vi "App - analyze RUS V6.vi"() -> ()   [LabVIEW 2015] (continued)
"z(0)"=0.0+0.0i, "radius"=0.0}}, "timestamp(min)"=2140.5666666701436, "timestamp"=timestamp(3493856255 s since 1904-01-01), "Magn Field(T)"=0.0}, {"temperature"=14.643, "lorentzian"={"Amplitude"=0.0, "omega(0)"=0.0, "Gamma"=0.0, "phase"=0.0, "Q"=0.0, "Norm  Ampl"=0.0, "z (inf)"=0.0+0.0i, "4corners"={"z (-pi/2)"=0.0+0.0i, "z(inf)"=0.0+0.0i, "z (pi/2)"=0.0+0.0i, "z center"=0.0+0.0i, "z(0)"=0.0+0.0i, "radius"=0.0}}, "timestamp(min)"=2141.89999999851, "timestamp"=timestamp(3493856335 s since 1904-01-01), "Magn Field(T)"=0.0}, {"temperature"=14.643, "lorentzian"={"Amplitude"=0.0, "omega(0)"=0.0, "Gamma"=0.0, "phase"=0.0, "Q"=0.0, "Norm  Ampl"=0.0, "z (inf)"=0.0+0.0i, "4corners"={"z (-pi/2)"=0.0+0.0i, "z(inf)"=0.0+0.0i, "z (pi/2)"=0.0+0.0i, "z center"=0.0+0.0i, "z(0)"=0.0+0.0i, "radius"=0.0}}, "timestamp(min)"=2143.2166666686535, "timestamp"=timestamp(3493856414 s since 1904-01-01), "Magn Field(T)"=0.0}, {"temperature"=14.638, "lorentzian"={"Amplitude"=0.0, "omega(0)"=0.0, "Gamma"=0.0, "phase"=0.0, "Q"=0.0, "Norm  Ampl"=0.0, "z (inf)"=0.0+0.0i, "4corners"={"z (-pi/2)"=0.0+0.0i, "z(inf)"=0.0+0.0i, "z (pi/2)"=0.0+0.0i, "z center"=0.0+0.0i, "z(0)"=0.0+0.0i, "radius"=0.0}}, "timestamp(min)"=2144.5333333313465, "timestamp"=timestamp(3493856493 s since 1904-01-01), "Magn Field(T)"=0.0}, {"temperature"=14.634, "lorentzian"={"Amplitude"=0.0, "omega(0)"=0.0, "Gamma"=0.0, "phase"=0.0, "Q"=0.0, "Norm  Ampl"=0.0, "z (inf)"=0.0+0.0i, "4corners"={"z (-pi/2)"=0.0+0.0i, "z(inf)"=0.0+0.0i, "z (pi/2)"=0.0+0.0i, "z center"=0.0+0.0i, "z(0)"=0.0+0.0i, "radius"=0.0}}, "timestamp(min)"=2145.8666666671634, "timestamp"=timestamp(3493856573 s since 1904-01-01), "Magn Field(T)"=0.0}, {"temperature"=14.63, "lorentzian"={"Amplitude"=0.0, "omega(0)"=0.0, "Gamma"=0.0, "phase"=0.0, "Q"=0.0, "Norm  Ampl"=0.0, "z (inf)"=0.0+0.0i, "4corners"={"z (-pi/2)"=0.0+0.0i, "z(inf)"=0.0+0.0i, "z (pi/2)"=0.0+0.0i, "z center"=0.0+0.0i, "z(0)"=0.0+0.0i, "radius"=0.0}}, "timestamp(min)"=2147.183333337307, "timestamp"=timestamp(3493856652 s since 1904-01-01), "Magn Field(T)"=0.0}, {"temperature"=14.628, "lorentzian"={"Amplitude"=0.0, "omega(0)"=0.0, "Gamma"=0.0, "phase"=0.0, "Q"=0.0, "Norm  Ampl"=0.0, "z (inf)"=0.0+0.0i, "4corners"={"z (-pi/2)"=0.0+0.0i, "z(inf)"=0.0+0.0i, "z (pi/2)"=0.0+0.0i, "z center"=0.0+0.0i, "z(0)"=0.0+0.0i, "radius"=0.0}}, "timestamp(min)"=2148.5166666656733, "timestamp"=timestamp(3493856732 s since 1904-01-01), "Magn Field(T)"=0.0}, {"temperature"=14.626, "lorentzian"={"Amplitude"=0.0, "omega(0)"=0.0, "Gamma"=0.0, "phase"=0.0, "Q"=0.0, "Norm  Ampl"=0.0, "z (inf)"=0.0+0.0i, "4corners"={"z (-pi/2)"=0.0+0.0i, "z(inf)"=0.0+0.0i, "z (pi/2)"=0.0+0.0i, "z center"=0.0+0.0i, "z(0)"=0.0+0.0i, "radius"=0.0}}, "timestamp(min)"=2149.833333335817, "timestamp"=timestamp(3493856811 s since 1904-01-01), "Magn Field(T)"=0.0}, {"temperature"=14.618, "lorentzian"={"Amplitude"=0.0, "omega(0)"=0.0, "Gamma"=0.0, "phase"=0.0, "Q"=0.0, "Norm  Ampl"=0.0, "z (inf)"=0.0+0.0i, "4corners"={"z (-pi/2)"=0.0+0.0i, "z(inf)"=0.0+0.0i, "z (pi/2)"=0.0+0.0i, "z center"=0.0+0.0i, "z(0)"=0.0+0.0i, "radius"=0.0}}, "timestamp(min)"=2151.14999999851, "timestamp"=timestamp(3493856890 s since 1904-01-01), "Magn Field(T)"=0.0}, {"temperature"=14.618, "lorentzian"={"Amplitude"=0.0, "omega(0)"=0.0, "Gamma"=0.0, "phase"=0.0, "Q"=0.0, "Norm  Ampl"=0.0, "z (inf)"=0.0+0.0i, "4corners"={"z (-pi/2)"=0.0+0.0i, "z(inf)"=0.0+0.0i, "z (pi/2)"=0.0+0.0i, "z center"=0.0+0.0i, "z(0)"=0.0+0.0i, "radius"=0.0}}, "timestamp(min)"=2152.4666666686535, "timestamp"=timestamp(3493856969 s since 1904-01-01), "Magn Field(T)"=0.0}, {"temperature"=14.621, "lorentzian"={"Amplitude"=0.0, "omega(0)"=0.0, "Gamma"=0.0, "phase"=0.0, "Q"=0.0, "Norm  Ampl"=0.0, "z (inf)"=0.0+0.0i, "4corners"={"z (-pi/2)"=0.0+0.0i, "z(inf)"=0.0+0.0i, "z (pi/2)"=0.0+0.0i, "z center"=0.0+0.0i, "z(0)"=0.0+0.0i, "radius"=0.0}}, "timestamp(min)"=2153.8000000044703, "timestamp"=timestamp(3493857049 s since 1904-01-01), "Magn Field(T)"=0.0}, {"temperature"=14.616, "lorentzian"={"Amplitude"=0.0, "omega(0)"=0.0, "Gamma"=0.0, "phase"=0.0, "Q"=0.0, "Norm  Ampl"=0.0, "z (inf)"=0.0+0.0i, "4corners"={"z (-pi/2)"=0.0+0.0i, "z(inf)"=0.0+0.0i, "z (pi/2)"=0.0+0.0i, "z center"=0.0+0.0i, "z(0)"=0.0+0.0i, "radius"=0.0}}, "timestamp(min)"=2155.1166666671634, "timestamp"=timestamp(3493857128 s since 1904-01-01), "Magn Field(T)"=0.0}, {"temperature"=14.612, "lorentzian"={"Amplitude"=0.0, "omega(0)"=0.0, "Gamma"=0.0, "phase"=0.0, "Q"=0.0, "Norm  Ampl"=0.0, "z (inf)"=0.0+0.0i, "4corners"={"z (-pi/2)"=0.0+0.0i, "z(inf)"=0.0+0.0i, "z (pi/2)"=0.0+0.0i, "z center"=0.0+0.0i, "z(0)"=0.0+0.0i, "radius"=0.0}}, "timestamp(min)"=2156.433333337307, "timestamp"=timestamp(3493857207 s since 1904-01-01), "Magn Field(T)"=0.0}, {"temperature"=14.606, "lorentzian"={"Amplitude"=0.0, "omega(0)"=0.0, "Gamma"=0.0, "phase"=0.0, "Q"=0.0, "Norm  Ampl"=0.0, "z (inf)"=0.0+0.0i, "4corners"={"z (-pi/2)"=0.0+0.0i, "z(inf)"=0.0+0.0i, "z (pi/2)"=0.0+0.0i, "z center"=0.0+0.0i, "z(0)"=0.0+0.0i, "radius"=0.0}}, "timestamp(min)"=2157.75, "timestamp"=timestamp(3493857286 s since 1904-01-01), "Magn Field(T)"=0.0}, {"temperature"=14.604, "lorentzian"={"Amplitude"=0.0, "omega(0)"=0.0, "Gamma"=0.0, "phase"=0.0, "Q"=0.0, "Norm  Ampl"=0.0, "z (inf)"=0.0+0.0i, "4corners"={"z (-pi/2)"=0.0+0.0i, "z(inf)"=0.0+0.0i, "z (pi/2)"=0.0+0.0i, "z center"=0.0+0.0i, "z(0)"=0.0+0.0i, "radius"=0.0}}, "timestamp(min)"=2159.083333335817, "timestamp"=timestamp(3493857366 s since 1904-01-01), "Magn Field(T)"=0.0}, {"temperature"=14.604, "lorentzian"={"Amplitude"=0.0, "omega(0)"=0.0, "Gamma"=0.0, "phase"=0.0, "Q"=0.0, "Norm  Ampl"=0.0, "z (inf)"=0.0+0.0i, "4corners"={"z (-pi/2)"=0.0+0.0i, "z(inf)"=0.0+0.0i, "z (pi/2)"=0.0+0.0i, "z center"=0.0+0.0i, "z(0)"=0.0+0.0i, "radius"=0.0}}, "timestamp(min)"=2160.39999999851, "timestamp"=timestamp(3493857445 s since 1904-01-01), "Magn Field(T)"=0.0}, {"temperature"=14.606, "lorentzian"={"Amplitude"=0.0, "omega(0)"=0.0, "Gamma"=0.0, "phase"=0.0, "Q"=0.0, "Norm  Ampl"=0.0, "z (inf)"=0.0+0.0i, "4corners"={"z (-pi/2)"=0.0+0.0i, "z(inf)"=0.0+0.0i, "z (pi/2)"=0.0+0.0i, "z center"=0.0+0.0i, "z(0)"=0.0+0.0i, "radius"=0.0}}, "timestamp(min)"=2161.7166666686535, "timestamp"=timestamp(3493857524 s since 1904-01-01), "Magn Field(T)"=0.0}, {"temperature"=14.605, "lorentzian"={"Amplitude"=0.0, "omega(0)"=0.0, "Gamma"=0.0, "phase"=0.0, "Q"=0.0, "Norm  Ampl"=0.0, "z (inf)"=0.0+0.0i, "4corners"={"z (-pi/2)"=0.0+0.0i, "z(inf)"=0.0+0.0i, "z (pi/2)"=0.0+0.0i, "z center"=0.0+0.0i, "z(0)"=0.0+0.0i, "radius"=0.0}}, "timestamp(min)"=2163.0500000044703, "timestamp"=timestamp(3493857604 s since 1904-01-01), "Magn Field(T)"=0.0}, {"temperature"=14.606, "lorentzian"={"Amplitude"=0.0, "omega(0)"=0.0, "Gamma"=0.0, "phase"=0.0, "Q"=0.0, "Norm  Ampl"=0.0, "z (inf)"=0.0+0.0i, "4corners"={"z (-pi/2)"=0.0+0.0i, "z(inf)"=0.0+0.0i, "z (pi/2)"=0.0+0.0i, "z center"=0.0+0.0i, "z(0)"=0.0+0.0i, "radius"=0.0}}, "timestamp(min)"=2164.3666666671634, "timestamp"=timestamp(3493857683 s since 1904-01-01), "Magn Field(T)"=0.0}, {"temperature"=14.603, "lorentzian"={"Amplitude"=0.0, "omega(0)"=0.0, "Gamma"=0.0, "phase"=0.0, "Q"=0.0, "Norm  Ampl"=0.0, "z (inf)"=0.0+0.0i, "4corners"={"z (-pi/2)"=0.0+0.0i, "z(inf)"=0.0+0.0i, "z (pi/2)"=0.0+0.0i, "z center"=0.0+0.0i, "z(0)"=0.0+0.0i, "radius"=0.0}}, "timestamp(min)"=2165.683333337307, "timestamp"=timestamp(3493857762 s since 1904-01-01), "Magn Field(T)"=0.0}, {"temperature"=14.6, "lorentzian"={"Amplitude"=0.0, "omega(0)"=0.0, "Gamma"=0.0, "phase"=0.0, "Q"=0.0, "Norm  Ampl"=0.0, "z (inf)"=0.0+0.0i, "4corners"={"z (-pi/2)"=0.0+0.0i, "z(inf)"=0.0+0.0i, "z (pi/2)"=0.0+0.0i, "z center"=0.0+0.0i, "z(0)"=0.0+0.0i, "radius"=0.0}}, "timestamp(min)"=2167.0166666656733, "timestamp"=timestamp(3493857842 s since 1904-01-01), "Magn Field(T)"=0.0}, {"temperature"=14.601, "lorentzian"={"Amplitude"=0.0, "omega(0)"=0.0, "Gamma"=0.0, "phase"=0.0, "Q"=0.0, "Norm  Ampl"=0.0, "z (inf)"=0.0+0.0i, "4corners"={"z (-pi/2)"=0.0+0.0i, "z(inf)"=0.0+0.0i, "z (pi/2)"=0.0+0.0i, "z center"=0.0+0.0i, "z(0)"=0.0+0.0i, "radius"=0.0}}, "timestamp(min)"=2168.333333335817, "timestamp"=timestamp(3493857921 s since 1904-01-01), "Magn Field(T)"=0.0}, {"temperature"=14.595, "lorentzian"={"Amplitude"=0.0, "omega(0)"=0.0, "Gamma"=0.0, "phase"=0.0, "Q"=0.0, "Norm  Ampl"=0.0, "z (inf)"=0.0+0.0i, "4corners"={"z (-pi/2)"=0.0+0.0i, "z(inf)"=0.0+0.0i, "z (pi/2)"=0.0+0.0i, "z center"=0.0+0.0i, "z(0)"=0.0+0.0i, "radius"=0.0}}, "timestamp(min)"=2169.64999999851, "timestamp"=timestamp(3493858000 s since 1904-01-01), "Magn Field(T)"=0.0}, {"temperature"=14.592, "lorentzian"={"Amplitude"=0.0, "omega(0)"=0.0, "Gamma"=0.0, "phase"=0.0, "Q"=0.0, "Norm  Ampl"=0.0, "z (inf)"=0.0+0.0i, "4corners"={"z (-pi/2)"=0.0+0.0i, "z(inf)"=0.0+0.0i, "z (pi/2)"=0.0+0.0i, "z center"=0.0+0.0i, "z(0)"=0.0+0.0i, "radius"=0.0}}, "timestamp(min)"=2170.9833333343267, "timestamp"=timestamp(3493858080 s since 1904-01-01), "Magn Field(T)"=0.0}, {"temperature"=14.59, "lorentzian"={"Amplitude"=0.0, "omega(0)"=0.0, "Gamma"=0.0, "phase"=0.0, "Q"=0.0, "Norm  Ampl"=0.0, "z (inf)"=0.0+0.0i, "4corners"={"z (-pi/2)"=0.0+0.0i, "z(inf)"=0.0+0.0i, "z (pi/2)"=0.0+0.0i, "z center"=0.0+0.0i, "z(0)"=0.0+0.0i, "radius"=0.0}}, "timestamp(min)"=2172.3000000044703, "timestamp"=timestamp(3493858159 s since 1904-01-01), "Magn Field(T)"=0.0}, {"temperature"=14.588, "lorentzian"={"Amplitude"=0.0, "omega(0)"=0.0, "Gamma"=0.0, "phase"=0.0, "Q"=0.0, "Norm  Ampl"=0.0, "z (inf)"=0.0+0.0i, "4corners"={"z (-pi/2)"=0.0+0.0i, "z(inf)"=0.0+0.0i, "z (pi/2)"=0.0+0.0i, "z center"=0.0+0.0i, "z(0)"=0.0+0.0i, "radius"=0.0}}, "timestamp(min)"=2173.6166666671634, "timestamp"=timestamp(3493858238 s since 1904-01-01), "Magn Field(T)"=0.0}, {"temperature"=14.586, "lorentzian"={"Amplitude"=0.0, "omega(0)"=0.0, "Gamma"=0.0, "phase"=0.0, "Q"=0.0, "Norm  Ampl"=0.0, "z (inf)"=0.0+0.0i, "4corners"={"z (-pi/2)"=0.0+0.0i, "z(inf)"=0.0+0.0i, "z (pi/2)"=0.0+0.0i, "z center"=0.0+0.0i, "z(0)"=0.0+0.0i, "radius"=0.0}}, "timestamp(min)"=2174.9500000029802, "timestamp"=timestamp(3493858318 s since 1904-01-01), "Magn Field(T)"=0.0}, {"temperature"=14.583, "lorentzian"={"Amplitude"=0.0, "omega(0)"=0.0, "Gamma"=0.0, "phase"=0.0, "Q"=0.0, "Norm  Ampl"=0.0, "z (inf)"=0.0+0.0i, "4corners"={"z (-pi/2)"=0.0+0.0i, "z(inf)"=0.0+0.0i, "z (pi/2)"=0.0+0.0i, "z center"=0.0+0.0i, "z(0)"=0.0+0.0i, "radius"=0.0}}, "timestamp(min)"=2176.2666666656733, "timestamp"=timestamp(3493858397 s since 1904-01-01), "Magn Field(T)"=0.0}, {"temperature"=14.577, "lorentzian"={"Amplitude"=0.0, "omega(0)"=0.0, "Gamma"=0.0, "phase"=0.0, "Q"=0.0, "Norm  Ampl"=0.0, "z (inf)"=0.0+0.0i, "4corners"={"z (-pi/2)"=0.0+0.0i, "z(inf)"=0.0+0.0i, "z (pi/2)"=0.0+0.0i, "z center"=0.0+0.0i, "z(0)"=0.0+0.0i, "radius"=0.0}}, "timestamp(min)"=2177.60000000149, "timestamp"=timestamp(3493858477 s since 1904-01-01), "Magn Field(T)"=0.0}, {"temperature"=14.575, "lorentzian"={"Amplitude"=0.0, "omega(0)"=0.0, "Gamma"=0.0, "phase"=0.0, "Q"=0.0, "Norm  Ampl"=0.0, "z (inf)"=0.0+0.0i, "4corners"={"z (-pi/2)"=0.0+0.0i, "z(inf)"=0.0+0.0i, "z (pi/2)"=0.0+0.0i, "z center"=0.0+0.0i, "z(0)"=0.0+0.0i, "radius"=0.0}}, "timestamp(min)"=2178.916666664183, "timestamp"=timestamp(3493858556 s since 1904-01-01), "Magn Field(T)"=0.0}, {"temperature"=14.575, "lorentzian"={"Amplitude"=0.0, "omega(0)"=0.0, "Gamma"=0.0, "phase"=0.0, "Q"=0.0, "Norm  Ampl"=0.0, "z (inf)"=0.0+0.0i, "4corners"={"z (-pi/2)"=0.0+0.0i, "z(inf)"=0.0+0.0i, "z (pi/2)"=0.0+0.0i, "z center"=0.0+0.0i, "z(0)"=0.0+0.0i, "radius"=0.0}}, "timestamp(min)"=2180.2333333343267, "timestamp"=timestamp(3493858635 s since 1904-01-01), "Magn Field(T)"=0.0}, {"temperature"=14.572, "lorentzian"={"Amplitude"=0.0, "omega(0)"=0.0, "Gamma"=0.0, "phase"=0.0, "Q"=0.0, "Norm  Ampl"=0.0, "z (inf)"=0.0+0.0i, "4corners"={"z (-pi/2)"=0.0+0.0i, "z(inf)"=0.0+0.0i, "z (pi/2)"=0.0+0.0i, "z center"=0.0+0.0i, "z(0)"=0.0+0.0i, "radius"=0.0}}, "timestamp(min)"=2181.5666666701436, "timestamp"=timestamp(3493858715 s since 1904-01-01), "Magn Field(T)"=0.0}, {"temperature"=14.574, "lorentzian"={"Amplitude"=0.0, "omega(0)"=0.0, "Gamma"=0.0, "phase"=0.0, "Q"=0.0, "Norm  Ampl"=0.0, "z (inf)"=0.0+0.0i, "4corners"={"z (-pi/2)"=0.0+0.0i, "z(inf)"=0.0+0.0i, "z (pi/2)"=0.0+0.0i, "z center"=0.0+0.0i, "z(0)"=0.0+0.0i, "radius"=0.0}}, "timestamp(min)"=2182.8833333328366, "timestamp"=timestamp(3493858794 s since 1904-01-01), "Magn Field(T)"=0.0}, {"temperature"=14.57, "lorentzian"={"Amplitude"=0.0, "omega(0)"=0.0, "Gamma"=0.0, "phase"=0.0, "Q"=0.0, "Norm  Ampl"=0.0, "z (inf)"=0.0+0.0i, "4corners"={"z (-pi/2)"=0.0+0.0i, "z(inf)"=0.0+0.0i, "z (pi/2)"=0.0+0.0i, "z center"=0.0+0.0i, "z(0)"=0.0+0.0i, "radius"=0.0}}, "timestamp(min)"=2184.2000000029802, "timestamp"=timestamp(3493858873 s since 1904-01-01), "Magn Field(T)"=0.0}, {"temperature"=14.574, "lorentzian"={"Amplitude"=0.0, "omega(0)"=0.0, "Gamma"=0.0, "phase"=0.0, "Q"=0.0, "Norm  Ampl"=0.0, "z (inf)"=0.0+0.0i, "4corners"={"z (-pi/2)"=0.0+0.0i, "z(inf)"=0.0+0.0i, "z (pi/2)"=0.0+0.0i, "z center"=0.0+0.0i, "z(0)"=0.0+0.0i, "radius"=0.0}}, "timestamp(min)"=2185.5333333313465, "timestamp"=timestamp(3493858953 s since 1904-01-01), "Magn Field(T)"=0.0}, {"temperature"=14.576, "lorentzian"={"Amplitude"=0.0, "omega(0)"=0.0, "Gamma"=0.0, "phase"=0.0, "Q"=0.0, "Norm  Ampl"=0.0, "z (inf)"=0.0+0.0i, "4corners"={"z (-pi/2)"=0.0+0.0i, "z(inf)"=0.0+0.0i, "z (pi/2)"=0.0+0.0i, "z center"=0.0+0.0i, "z(0)"=0.0+0.0i, "radius"=0.0}}, "timestamp(min)"=2186.85000000149, "timestamp"=timestamp(3493859032 s since 1904-01-01), "Magn Field(T)"=0.0}, {"temperature"=14.575, "lorentzian"={"Amplitude"=0.0, "omega(0)"=0.0, "Gamma"=0.0, "phase"=0.0, "Q"=0.0, "Norm  Ampl"=0.0, "z (inf)"=0.0+0.0i, "4corners"={"z (-pi/2)"=0.0+0.0i, "z(inf)"=0.0+0.0i, "z (pi/2)"=0.0+0.0i, "z center"=0.0+0.0i, "z(0)"=0.0+0.0i, "radius"=0.0}}, "timestamp(min)"=2188.183333337307, "timestamp"=timestamp(3493859112 s since 1904-01-01), "Magn Field(T)"=0.0}, {"temperature"=14.567, "lorentzian"={"Amplitude"=0.0, "omega(0)"=0.0, "Gamma"=0.0, "phase"=0.0, "Q"=0.0, "Norm  Ampl"=0.0, "z (inf)"=0.0+0.0i, "4corners"={"z (-pi/2)"=0.0+0.0i, "z(inf)"=0.0+0.0i, "z (pi/2)"=0.0+0.0i, "z center"=0.0+0.0i, "z(0)"=0.0+0.0i, "radius"=0.0}}, "timestamp(min)"=2189.5, "timestamp"=timestamp(3493859191 s since 1904-01-01), "Magn Field(T)"=0.0}, {"temperature"=14.572, "lorentzian"={"Amplitude"=0.0, "omega(0)"=0.0, "Gamma"=0.0, "phase"=0.0, "Q"=0.0, "Norm  Ampl"=0.0, "z (inf)"=0.0+0.0i, "4corners"={"z (-pi/2)"=0.0+0.0i, "z(inf)"=0.0+0.0i, "z (pi/2)"=0.0+0.0i, "z center"=0.0+0.0i, "z(0)"=0.0+0.0i, "radius"=0.0}}, "timestamp(min)"=2190.8166666701436, "timestamp"=timestamp(3493859270 s since 1904-01-01), "Magn Field(T)"=0.0}, {"temperature"=14.571, "lorentzian"={"Amplitude"=0.0, "omega(0)"=0.0, "Gamma"=0.0, "phase"=0.0, "Q"=0.0, "Norm  Ampl"=0.0, "z (inf)"=0.0+0.0i, "4corners"={"z (-pi/2)"=0.0+0.0i, "z(inf)"=0.0+0.0i, "z (pi/2)"=0.0+0.0i, "z center"=0.0+0.0i, "z(0)"=0.0+0.0i, "radius"=0.0}}, "timestamp(min)"=2192.14999999851, "timestamp"=timestamp(3493859350 s since 1904-01-01), "Magn Field(T)"=0.0}, {"temperature"=14.568, "lorentzian"={"Amplitude"=0.0, "omega(0)"=0.0, "Gamma"=0.0, "phase"=0.0, "Q"=0.0, "Norm  Ampl"=0.0, "z (inf)"=0.0+0.0i, "4corners"={"z (-pi/2)"=0.0+0.0i, "z(inf)"=0.0+0.0i, "z (pi/2)"=0.0+0.0i, "z center"=0.0+0.0i, "z(0)"=0.0+0.0i, "radius"=0.0}}, "timestamp(min)"=2193.4666666686535, "timestamp"=timestamp(3493859429 s since 1904-01-01), "Magn Field(T)"=0.0}, {"temperature"=14.564, "lorentzian"={"Amplitude"=0.0, "omega(0)"=0.0, "Gamma"=0.0, "phase"=0.0, "Q"=0.0, "Norm  Ampl"=0.0, "z (inf)"=0.0+0.0i, "4corners"={"z (-pi/2)"=0.0+0.0i, "z(inf)"=0.0+0.0i, "z (pi/2)"=0.0+0.0i, "z center"=0.0+0.0i, "z(0)"=0.0+0.0i, "radius"=0.0}}, "timestamp(min)"=2194.7833333313465, "timestamp"=timestamp(3493859508 s since 1904-01-01), "Magn Field(T)"=0.0}, {"temperature"=14.565, "lorentzian"={"Amplitude"=0.0, "omega(0)"=0.0, "Gamma"=0.0, "phase"=0.0, "Q"=0.0, "Norm  Ampl"=0.0, "z (inf)"=0.0+0.0i, "4corners"={"z (-pi/2)"=0.0+0.0i, "z(inf)"=0.0+0.0i, "z (pi/2)"=0.0+0.0i, "z center"=0.0+0.0i, "z(0)"=0.0+0.0i, "radius"=0.0}}, "timestamp(min)"=2196.1166666671634, "timestamp"=timestamp(3493859588 s since 1904-01-01), "Magn Field(T)"=0.0}, {"temperature"=14.561, "lorentzian"={"Amplitude"=0.0, "omega(0)"=0.0, "Gamma"=0.0, "phase"=0.0, "Q"=0.0, "Norm  Ampl"=0.0, "z (inf)"=0.0+0.0i, "4corners"={"z (-pi/2)"=0.0+0.0i, "z(inf)"=0.0+0.0i, "z (pi/2)"=0.0+0.0i, "z center"=0.0+0.0i, "z(0)"=0.0+0.0i, "radius"=0.0}}, "timestamp(min)"=2197.433333337307, "timestamp"=timestamp(3493859667 s since 1904-01-01), "Magn Field(T)"=0.0}, {"temperature"=14.557, "lorentzian"={"Amplitude"=0.0, "omega(0)"=0.0, "Gamma"=0.0, "phase"=0.0, "Q"=0.0, "Norm  Ampl"=0.0, "z (inf)"=0.0+0.0i, "4corners"={"z (-pi/2)"=0.0+0.0i, "z(inf)"=0.0+0.0i, "z (pi/2)"=0.0+0.0i, "z center"=0.0+0.0i, "z(0)"=0.0+0.0i, "radius"=0.0}}, "timestamp(min)"=2198.7666666656733, "timestamp"=timestamp(3493859747 s since 1904-01-01), "Magn Field(T)"=0.0}, {"temperature"=14.553, "lorentzian"={"Amplitude"=0.0, "omega(0)"=0.0, "Gamma"=0.0, "phase"=0.0, "Q"=0.0, "Norm  Ampl"=0.0, "z (inf)"=0.0+0.0i, "4corners"={"z (-pi/2)"=0.0+0.0i, "z(inf)"=0.0+0.0i, "z (pi/2)"=0.0+0.0i, "z center"=0.0+0.0i, "z(0)"=0.0+0.0i, "radius"=0.0}}, "timestamp(min)"=2200.083333335817, "timestamp"=timestamp(3493859826 s since 1904-01-01), "Magn Field(T)"=0.0}, {"temperature"=14.55, "lorentzian"={"Amplitude"=0.0, "omega(0)"=0.0, "Gamma"=0.0, "phase"=0.0, "Q"=0.0, "Norm  Ampl"=0.0, "z (inf)"=0.0+0.0i, "4corners"={"z (-pi/2)"=0.0+0.0i, "z(inf)"=0.0+0.0i, "z (pi/2)"=0.0+0.0i, "z center"=0.0+0.0i, "z(0)"=0.0+0.0i, "radius"=0.0}}, "timestamp(min)"=2201.39999999851, "timestamp"=timestamp(3493859905 s since 1904-01-01), "Magn Field(T)"=0.0}, {"temperature"=14.546, "lorentzian"={"Amplitude"=0.0, "omega(0)"=0.0, "Gamma"=0.0, "phase"=0.0, "Q"=0.0, "Norm  Ampl"=0.0, "z (inf)"=0.0+0.0i, "4corners"={"z (-pi/2)"=0.0+0.0i, "z(inf)"=0.0+0.0i, "z (pi/2)"=0.0+0.0i, "z center"=0.0+0.0i, "z(0)"=0.0+0.0i, "radius"=0.0}}, "timestamp(min)"=2202.7333333343267, "timestamp"=timestamp(3493859985 s since 1904-01-01), "Magn Field(T)"=0.0}, {"temperature"=14.543, "lorentzian"={"Amplitude"=0.0, "omega(0)"=0.0, "Gamma"=0.0, "phase"=0.0, "Q"=0.0, "Norm  Ampl"=0.0, "z (inf)"=0.0+0.0i, "4corners"={"z (-pi/2)"=0.0+0.0i, "z(inf)"=0.0+0.0i, "z (pi/2)"=0.0+0.0i, "z center"=0.0+0.0i, "z(0)"=0.0+0.0i, "radius"=0.0}}, "timestamp(min)"=2204.0500000044703, "timestamp"=timestamp(3493860064 s since 1904-01-01), "Magn Field(T)"=0.0}, {"temperature"=14.545, "lorentzian"={"Amplitude"=0.0, "omega(0)"=0.0, "Gamma"=0.0, "phase"=0.0, "Q"=0.0, "Norm  Ampl"=0.0, "z (inf)"=0.0+0.0i, "4corners"={"z (-pi/2)"=0.0+0.0i, "z(inf)"=0.0+0.0i, "z (pi/2)"=0.0+0.0i, "z center"=0.0+0.0i, "z(0)"=0.0+0.0i, "radius"=0.0}}, "timestamp(min)"=2205.3833333328366, "timestamp"=timestamp(3493860144 s since 1904-01-01), "Magn Field(T)"=0.0}, {"temperature"=14.546, "lorentzian"={"Amplitude"=0.0, "omega(0)"=0.0, "Gamma"=0.0, "phase"=0.0, "Q"=0.0, "Norm  Ampl"=0.0, "z (inf)"=0.0+0.0i, "4corners"={"z (-pi/2)"=0.0+0.0i, "z(inf)"=0.0+0.0i, "z (pi/2)"=0.0+0.0i, "z center"=0.0+0.0i, "z(0)"=0.0+0.0i, "radius"=0.0}}, "timestamp(min)"=2206.7000000029802, "timestamp"=timestamp(3493860223 s since 1904-01-01), "Magn Field(T)"=0.0}, {"temperature"=14.542, "lorentzian"={"Amplitude"=0.0, "omega(0)"=0.0, "Gamma"=0.0, "phase"=0.0, "Q"=0.0, "Norm  Ampl"=0.0, "z (inf)"=0.0+0.0i, "4corners"={"z (-pi/2)"=0.0+0.0i, "z(inf)"=0.0+0.0i, "z (pi/2)"=0.0+0.0i, "z center"=0.0+0.0i, "z(0)"=0.0+0.0i, "radius"=0.0}}, "timestamp(min)"=2208.0166666656733, "timestamp"=timestamp(3493860302 s since 1904-01-01), "Magn Field(T)"=0.0}, {"temperature"=14.545, "lorentzian"={"Amplitude"=0.0, "omega(0)"=0.0, "Gamma"=0.0, "phase"=0.0, "Q"=0.0, "Norm  Ampl"=0.0, "z (inf)"=0.0+0.0i, "4corners"={"z (-pi/2)"=0.0+0.0i, "z(inf)"=0.0+0.0i, "z (pi/2)"=0.0+0.0i, "z center"=0.0+0.0i, "z(0)"=0.0+0.0i, "radius"=0.0}}, "timestamp(min)"=2209.35000000149, "timestamp"=timestamp(3493860382 s since 1904-01-01), "Magn Field(T)"=0.0}, {"temperature"=14.547, "lorentzian"={"Amplitude"=0.0, "omega(0)"=0.0, "Gamma"=0.0, "phase"=0.0, "Q"=0.0, "Norm  Ampl"=0.0, "z (inf)"=0.0+0.0i, "4corners"={"z (-pi/2)"=0.0+0.0i, "z(inf)"=0.0+0.0i, "z (pi/2)"=0.0+0.0i, "z center"=0.0+0.0i, "z(0)"=0.0+0.0i, "radius"=0.0}}, "timestamp(min)"=2210.666666664183, "timestamp"=timestamp(3493860461 s since 1904-01-01), "Magn Field(T)"=0.0}, {"temperature"=14.544, "lorentzian"={"Amplitude"=0.0, "omega(0)"=0.0, "Gamma"=0.0, "phase"=0.0, "Q"=0.0, "Norm  Ampl"=0.0, "z (inf)"=0.0+0.0i, "4corners"={"z (-pi/2)"=0.0+0.0i, "z(inf)"=0.0+0.0i, "z (pi/2)"=0.0+0.0i, "z center"=0.0+0.0i, "z(0)"=0.0+0.0i, "radius"=0.0}}, "timestamp(min)"=2211.9833333343267, "timestamp"=timestamp(3493860540 s since 1904-01-01), "Magn Field(T)"=0.0}, {"temperature"=14.538, "lorentzian"={"Amplitude"=0.0, "omega(0)"=0.0, "Gamma"=0.0, "phase"=0.0, "Q"=0.0, "Norm  Ampl"=0.0, "z (inf)"=0.0+0.0i, "4corners"={"z (-pi/2)"=0.0+0.0i, "z(inf)"=0.0+0.0i, "z (pi/2)"=0.0+0.0i, "z center"=0.0+0.0i, "z(0)"=0.0+0.0i, "radius"=0.0}}, "timestamp(min)"=2213.3166666701436, "timestamp"=timestamp(3493860620 s since 1904-01-01), "Magn Field(T)"=0.0}, {"temperature"=14.537, "lorentzian"={"Amplitude"=0.0, "omega(0)"=0.0, "Gamma"=0.0, "phase"=0.0, "Q"=0.0, "Norm  Ampl"=0.0, "z (inf)"=0.0+0.0i, "4corners"={"z (-pi/2)"=0.0+0.0i, "z(inf)"=0.0+0.0i, "z (pi/2)"=0.0+0.0i, "z center"=0.0+0.0i, "z(0)"=0.0+0.0i, "radius"=0.0}}, "timestamp(min)"=2214.6333333328366, "timestamp"=timestamp(3493860699 s since 1904-01-01), "Magn Field(T)"=0.0}, {"temperature"=14.527, "lorentzian"={"Amplitude"=0.0, "omega(0)"=0.0, "Gamma"=0.0, "phase"=0.0, "Q"=0.0, "Norm  Ampl"=0.0, "z (inf)"=0.0+0.0i, "4corners"={"z (-pi/2)"=0.0+0.0i, "z(inf)"=0.0+0.0i, "z (pi/2)"=0.0+0.0i, "z center"=0.0+0.0i, "z(0)"=0.0+0.0i, "radius"=0.0}}, "timestamp(min)"=2215.9666666686535, "timestamp"=timestamp(3493860779 s since 1904-01-01), "Magn Field(T)"=0.0}, {"temperature"=14.532, "lorentzian"={"Amplitude"=0.0, "omega(0)"=0.0, "Gamma"=0.0, "phase"=0.0, "Q"=0.0, "Norm  Ampl"=0.0, "z (inf)"=0.0+0.0i, "4corners"={"z (-pi/2)"=0.0+0.0i, "z(inf)"=0.0+0.0i, "z (pi/2)"=0.0+0.0i, "z center"=0.0+0.0i, "z(0)"=0.0+0.0i, "radius"=0.0}}, "timestamp(min)"=2217.2833333313465, "timestamp"=timestamp(3493860858 s since 1904-01-01), "Magn Field(T)"=0.0}, {"temperature"=14.532, "lorentzian"={"Amplitude"=0.0, "omega(0)"=0.0, "Gamma"=0.0, "phase"=0.0, "Q"=0.0, "Norm  Ampl"=0.0, "z (inf)"=0.0+0.0i, "4corners"={"z (-pi/2)"=0.0+0.0i, "z(inf)"=0.0+0.0i, "z (pi/2)"=0.0+0.0i, "z center"=0.0+0.0i, "z(0)"=0.0+0.0i, "radius"=0.0}}, "timestamp(min)"=2218.60000000149, "timestamp"=timestamp(3493860937 s since 1904-01-01), "Magn Field(T)"=0.0}, {"temperature"=14.525, "lorentzian"={"Amplitude"=0.0, "omega(0)"=0.0, "Gamma"=0.0, "phase"=0.0, "Q"=0.0, "Norm  Ampl"=0.0, "z (inf)"=0.0+0.0i, "4corners"={"z (-pi/2)"=0.0+0.0i, "z(inf)"=0.0+0.0i, "z (pi/2)"=0.0+0.0i, "z center"=0.0+0.0i, "z(0)"=0.0+0.0i, "radius"=0.0}}, "timestamp(min)"=2219.933333337307, "timestamp"=timestamp(3493861017 s since 1904-01-01), "Magn Field(T)"=0.0}, {"temperature"=14.52, "lorentzian"={"Amplitude"=0.0, "omega(0)"=0.0, "Gamma"=0.0, "phase"=0.0, "Q"=0.0, "Norm  Ampl"=0.0, "z (inf)"=0.0+0.0i, "4corners"={"z (-pi/2)"=0.0+0.0i, "z(inf)"=0.0+0.0i, "z (pi/2)"=0.0+0.0i, "z center"=0.0+0.0i, "z(0)"=0.0+0.0i, "radius"=0.0}}, "timestamp(min)"=2221.25, "timestamp"=timestamp(3493861096 s since 1904-01-01), "Magn Field(T)"=0.0}, {"temperature"=14.519, "lorentzian"={"Amplitude"=0.0, "omega(0)"=0.0, "Gamma"=0.0, "phase"=0.0, "Q"=0.0, "Norm  Ampl"=0.0, "z (inf)"=0.0+0.0i, "4corners"={"z (-pi/2)"=0.0+0.0i, "z(inf)"=0.0+0.0i, "z (pi/2)"=0.0+0.0i, "z center"=0.0+0.0i, "z(0)"=0.0+0.0i, "radius"=0.0}}, "timestamp(min)"=2222.5666666701436, "timestamp"=timestamp(3493861175 s since 1904-01-01), "Magn Field(T)"=0.0}, {"temperature"=14.515, "lorentzian"={"Amplitude"=0.0, "omega(0)"=0.0, "Gamma"=0.0, "phase"=0.0, "Q"=0.0, "Norm  Ampl"=0.0, "z (inf)"=0.0+0.0i, "4corners"={"z (-pi/2)"=0.0+0.0i, "z(inf)"=0.0+0.0i, "z (pi/2)"=0.0+0.0i, "z center"=0.0+0.0i, "z(0)"=0.0+0.0i, "radius"=0.0}}, "timestamp(min)"=2223.89999999851, "timestamp"=timestamp(3493861255 s since 1904-01-01), "Magn Field(T)"=0.0}, {"temperature"=14.515, "lorentzian"={"Amplitude"=0.0, "omega(0)"=0.0, "Gamma"=0.0, "phase"=0.0, "Q"=0.0, "Norm  Ampl"=0.0, "z (inf)"=0.0+0.0i, "4corners"={"z (-pi/2)"=0.0+0.0i, "z(inf)"=0.0+0.0i, "z (pi/2)"=0.0+0.0i, "z center"=0.0+0.0i, "z(0)"=0.0+0.0i, "radius"=0.0}}, "timestamp(min)"=2225.2166666686535, "timestamp"=timestamp(3493861334 s since 1904-01-01), "Magn Field(T)"=0.0}, {"temperature"=14.511, "lorentzian"={"Amplitude"=0.0, "omega(0)"=0.0, "Gamma"=0.0, "phase"=0.0, "Q"=0.0, "Norm  Ampl"=0.0, "z (inf)"=0.0+0.0i, "4corners"={"z (-pi/2)"=0.0+0.0i, "z(inf)"=0.0+0.0i, "z (pi/2)"=0.0+0.0i, "z center"=0.0+0.0i, "z(0)"=0.0+0.0i, "radius"=0.0}}, "timestamp(min)"=2226.5500000044703, "timestamp"=timestamp(3493861414 s since 1904-01-01), "Magn Field(T)"=0.0}, {"temperature"=14.506, "lorentzian"={"Amplitude"=0.0, "omega(0)"=0.0, "Gamma"=0.0, "phase"=0.0, "Q"=0.0, "Norm  Ampl"=0.0, "z (inf)"=0.0+0.0i, "4corners"={"z (-pi/2)"=0.0+0.0i, "z(inf)"=0.0+0.0i, "z (pi/2)"=0.0+0.0i, "z center"=0.0+0.0i, "z(0)"=0.0+0.0i, "radius"=0.0}}, "timestamp(min)"=2227.8666666671634, "timestamp"=timestamp(3493861493 s since 1904-01-01), "Magn Field(T)"=0.0}, {"temperature"=14.507, "lorentzian"={"Amplitude"=0.0, "omega(0)"=0.0, "Gamma"=0.0, "phase"=0.0, "Q"=0.0, "Norm  Ampl"=0.0, "z (inf)"=0.0+0.0i, "4corners"={"z (-pi/2)"=0.0+0.0i, "z(inf)"=0.0+0.0i, "z (pi/2)"=0.0+0.0i, "z center"=0.0+0.0i, "z(0)"=0.0+0.0i, "radius"=0.0}}, "timestamp(min)"=2229.183333337307, "timestamp"=timestamp(3493861572 s since 1904-01-01), "Magn Field(T)"=0.0}, {"temperature"=14.503, "lorentzian"={"Amplitude"=0.0, "omega(0)"=0.0, "Gamma"=0.0, "phase"=0.0, "Q"=0.0, "Norm  Ampl"=0.0, "z (inf)"=0.0+0.0i, "4corners"={"z (-pi/2)"=0.0+0.0i, "z(inf)"=0.0+0.0i, "z (pi/2)"=0.0+0.0i, "z center"=0.0+0.0i, "z(0)"=0.0+0.0i, "radius"=0.0}}, "timestamp(min)"=2230.5166666656733, "timestamp"=timestamp(3493861652 s since 1904-01-01), "Magn Field(T)"=0.0}, {"temperature"=14.501, "lorentzian"={"Amplitude"=0.0, "omega(0)"=0.0, "Gamma"=0.0, "phase"=0.0, "Q"=0.0, "Norm  Ampl"=0.0, "z (inf)"=0.0+0.0i, "4corners"={"z (-pi/2)"=0.0+0.0i, "z(inf)"=0.0+0.0i, "z (pi/2)"=0.0+0.0i, "z center"=0.0+0.0i, "z(0)"=0.0+0.0i, "radius"=0.0}}, "timestamp(min)"=2231.833333335817, "timestamp"=timestamp(3493861731 s since 1904-01-01), "Magn Field(T)"=0.0}, {"temperature"=14.5, "lorentzian"={"Amplitude"=0.0, "omega(0)"=0.0, "Gamma"=0.0, "phase"=0.0, "Q"=0.0, "Norm  Ampl"=0.0, "z (inf)"=0.0+0.0i, "4corners"={"z (-pi/2)"=0.0+0.0i, "z(inf)"=0.0+0.0i, "z (pi/2)"=0.0+0.0i, "z center"=0.0+0.0i, "z(0)"=0.0+0.0i, "radius"=0.0}}, "timestamp(min)"=2233.166666664183, "timestamp"=timestamp(3493861811 s since 1904-01-01), "Magn Field(T)"=0.0}, {"temperature"=14.504, "lorentzian"={"Amplitude"=0.0, "omega(0)"=0.0, "Gamma"=0.0, "phase"=0.0, "Q"=0.0, "Norm  Ampl"=0.0, "z (inf)"=0.0+0.0i, "4corners"={"z (-pi/2)"=0.0+0.0i, "z(inf)"=0.0+0.0i, "z (pi/2)"=0.0+0.0i, "z center"=0.0+0.0i, "z(0)"=0.0+0.0i, "radius"=0.0}}, "timestamp(min)"=2234.4833333343267, "timestamp"=timestamp(3493861890 s since 1904-01-01), "Magn Field(T)"=0.0}, {"temperature"=14.504, "lorentzian"={"Amplitude"=0.0, "omega(0)"=0.0, "Gamma"=0.0, "phase"=0.0, "Q"=0.0, "Norm  Ampl"=0.0, "z (inf)"=0.0+0.0i, "4corners"={"z (-pi/2)"=0.0+0.0i, "z(inf)"=0.0+0.0i, "z (pi/2)"=0.0+0.0i, "z center"=0.0+0.0i, "z(0)"=0.0+0.0i, "radius"=0.0}}, "timestamp(min)"=2235.8000000044703, "timestamp"=timestamp(3493861969 s since 1904-01-01), "Magn Field(T)"=0.0}, {"temperature"=14.507, "lorentzian"={"Amplitude"=0.0, "omega(0)"=0.0, "Gamma"=0.0, "phase"=0.0, "Q"=0.0, "Norm  Ampl"=0.0, "z (inf)"=0.0+0.0i, "4corners"={"z (-pi/2)"=0.0+0.0i, "z(inf)"=0.0+0.0i, "z (pi/2)"=0.0+0.0i, "z center"=0.0+0.0i, "z(0)"=0.0+0.0i, "radius"=0.0}}, "timestamp(min)"=2237.1333333328366, "timestamp"=timestamp(3493862049 s since 1904-01-01), "Magn Field(T)"=0.0}, {"temperature"=14.502, "lorentzian"={"Amplitude"=0.0, "omega(0)"=0.0, "Gamma"=0.0, "phase"=0.0, "Q"=0.0, "Norm  Ampl"=0.0, "z (inf)"=0.0+0.0i, "4corners"={"z (-pi/2)"=0.0+0.0i, "z(inf)"=0.0+0.0i, "z (pi/2)"=0.0+0.0i, "z center"=0.0+0.0i, "z(0)"=0.0+0.0i, "radius"=0.0}}, "timestamp(min)"=2238.4500000029802, "timestamp"=timestamp(3493862128 s since 1904-01-01), "Magn Field(T)"=0.0}, {"temperature"=14.501, "lorentzian"={"Amplitude"=0.0, "omega(0)"=0.0, "Gamma"=0.0, "phase"=0.0, "Q"=0.0, "Norm  Ampl"=0.0, "z (inf)"=0.0+0.0i, "4corners"={"z (-pi/2)"=0.0+0.0i, "z(inf)"=0.0+0.0i, "z (pi/2)"=0.0+0.0i, "z center"=0.0+0.0i, "z(0)"=0.0+0.0i, "radius"=0.0}}, "timestamp(min)"=2239.7666666656733, "timestamp"=timestamp(3493862207 s since 1904-01-01), "Magn Field(T)"=0.0}, {"temperature"=14.503, "lorentzian"={"Amplitude"=0.0, "omega(0)"=0.0, "Gamma"=0.0, "phase"=0.0, "Q"=0.0, "Norm  Ampl"=0.0, "z (inf)"=0.0+0.0i, "4corners"={"z (-pi/2)"=0.0+0.0i, "z(inf)"=0.0+0.0i, "z (pi/2)"=0.0+0.0i, "z center"=0.0+0.0i, "z(0)"=0.0+0.0i, "radius"=0.0}}, "timestamp(min)"=2241.10000000149, "timestamp"=timestamp(3493862287 s since 1904-01-01), "Magn Field(T)"=0.0}, {"temperature"=14.496, "lorentzian"={"Amplitude"=0.0, "omega(0)"=0.0, "Gamma"=0.0, "phase"=0.0, "Q"=0.0, "Norm  Ampl"=0.0, "z (inf)"=0.0+0.0i, "4corners"={"z (-pi/2)"=0.0+0.0i, "z(inf)"=0.0+0.0i, "z (pi/2)"=0.0+0.0i, "z center"=0.0+0.0i, "z(0)"=0.0+0.0i, "radius"=0.0}}, "timestamp(min)"=2242.416666664183, "timestamp"=timestamp(3493862366 s since 1904-01-01), "Magn Field(T)"=0.0}, {"temperature"=14.494, "lorentzian"={"Amplitude"=0.0, "omega(0)"=0.0, "Gamma"=0.0, "phase"=0.0, "Q"=0.0, "Norm  Ampl"=0.0, "z (inf)"=0.0+0.0i, "4corners"={"z (-pi/2)"=0.0+0.0i, "z(inf)"=0.0+0.0i, "z (pi/2)"=0.0+0.0i, "z center"=0.0+0.0i, "z(0)"=0.0+0.0i, "radius"=0.0}}, "timestamp(min)"=2243.75, "timestamp"=timestamp(3493862446 s since 1904-01-01), "Magn Field(T)"=0.0}, {"temperature"=14.494, "lorentzian"={"Amplitude"=0.0, "omega(0)"=0.0, "Gamma"=0.0, "phase"=0.0, "Q"=0.0, "Norm  Ampl"=0.0, "z (inf)"=0.0+0.0i, "4corners"={"z (-pi/2)"=0.0+0.0i, "z(inf)"=0.0+0.0i, "z (pi/2)"=0.0+0.0i, "z center"=0.0+0.0i, "z(0)"=0.0+0.0i, "radius"=0.0}}, "timestamp(min)"=2245.0666666701436, "timestamp"=timestamp(3493862525 s since 1904-01-01), "Magn Field(T)"=0.0}, {"temperature"=14.485, "lorentzian"={"Amplitude"=0.0, "omega(0)"=0.0, "Gamma"=0.0, "phase"=0.0, "Q"=0.0, "Norm  Ampl"=0.0, "z (inf)"=0.0+0.0i, "4corners"={"z (-pi/2)"=0.0+0.0i, "z(inf)"=0.0+0.0i, "z (pi/2)"=0.0+0.0i, "z center"=0.0+0.0i, "z(0)"=0.0+0.0i, "radius"=0.0}}, "timestamp(min)"=2246.3833333328366, "timestamp"=timestamp(3493862604 s since 1904-01-01), "Magn Field(T)"=0.0}, {"temperature"=14.485, "lorentzian"={"Amplitude"=0.0, "omega(0)"=0.0, "Gamma"=0.0, "phase"=0.0, "Q"=0.0, "Norm  Ampl"=0.0, "z (inf)"=0.0+0.0i, "4corners"={"z (-pi/2)"=0.0+0.0i, "z(inf)"=0.0+0.0i, "z (pi/2)"=0.0+0.0i, "z center"=0.0+0.0i, "z(0)"=0.0+0.0i, "radius"=0.0}}, "timestamp(min)"=2247.7166666686535, "timestamp"=timestamp(3493862684 s since 1904-01-01), "Magn Field(T)"=0.0}, {"temperature"=14.487, "lorentzian"={"Amplitude"=0.0, "omega(0)"=0.0, "Gamma"=0.0, "phase"=0.0, "Q"=0.0, "Norm  Ampl"=0.0, "z (inf)"=0.0+0.0i, "4corners"={"z (-pi/2)"=0.0+0.0i, "z(inf)"=0.0+0.0i, "z (pi/2)"=0.0+0.0i, "z center"=0.0+0.0i, "z(0)"=0.0+0.0i, "radius"=0.0}}, "timestamp(min)"=2249.0333333313465, "timestamp"=timestamp(3493862763 s since 1904-01-01), "Magn Field(T)"=0.0}, {"temperature"=14.486, "lorentzian"={"Amplitude"=0.0, "omega(0)"=0.0, "Gamma"=0.0, "phase"=0.0, "Q"=0.0, "Norm  Ampl"=0.0, "z (inf)"=0.0+0.0i, "4corners"={"z (-pi/2)"=0.0+0.0i, "z(inf)"=0.0+0.0i, "z (pi/2)"=0.0+0.0i, "z center"=0.0+0.0i, "z(0)"=0.0+0.0i, "radius"=0.0}}, "timestamp(min)"=2250.35000000149, "timestamp"=timestamp(3493862842 s since 1904-01-01), "Magn Field(T)"=0.0}, {"temperature"=14.479, "lorentzian"={"Amplitude"=0.0, "omega(0)"=0.0, "Gamma"=0.0, "phase"=0.0, "Q"=0.0, "Norm  Ampl"=0.0, "z (inf)"=0.0+0.0i, "4corners"={"z (-pi/2)"=0.0+0.0i, "z(inf)"=0.0+0.0i, "z (pi/2)"=0.0+0.0i, "z center"=0.0+0.0i, "z(0)"=0.0+0.0i, "radius"=0.0}}, "timestamp(min)"=2251.683333337307, "timestamp"=timestamp(3493862922 s since 1904-01-01), "Magn Field(T)"=0.0}, {"temperature"=14.477, "lorentzian"={"Amplitude"=0.0, "omega(0)"=0.0, "Gamma"=0.0, "phase"=0.0, "Q"=0.0, "Norm  Ampl"=0.0, "z (inf)"=0.0+0.0i, "4corners"={"z (-pi/2)"=0.0+0.0i, "z(inf)"=0.0+0.0i, "z (pi/2)"=0.0+0.0i, "z center"=0.0+0.0i, "z(0)"=0.0+0.0i, "radius"=0.0}}, "timestamp(min)"=2253.0, "timestamp"=timestamp(3493863001 s since 1904-01-01), "Magn Field(T)"=0.0}, {"temperature"=14.476, "lorentzian"={"Amplitude"=0.0, "omega(0)"=0.0, "Gamma"=0.0, "phase"=0.0, "Q"=0.0, "Norm  Ampl"=0.0, "z (inf)"=0.0+0.0i, "4corners"={"z (-pi/2)"=0.0+0.0i, "z(inf)"=0.0+0.0i, "z (pi/2)"=0.0+0.0i, "z center"=0.0+0.0i, "z(0)"=0.0+0.0i, "radius"=0.0}}, "timestamp(min)"=2254.333333335817, "timestamp"=timestamp(3493863081 s since 1904-01-01), "Magn Field(T)"=0.0}, {"temperature"=14.474, "lorentzian"={"Amplitude"=0.0, "omega(0)"=0.0, "Gamma"=0.0, "phase"=0.0, "Q"=0.0, "Norm  Ampl"=0.0, "z (inf)"=0.0+0.0i, "4corners"={"z (-pi/2)"=0.0+0.0i, "z(inf)"=0.0+0.0i, "z (pi/2)"=0.0+0.0i, "z center"=0.0+0.0i, "z(0)"=0.0+0.0i, "radius"=0.0}}, "timestamp(min)"=2255.64999999851, "timestamp"=timestamp(3493863160 s since 1904-01-01), "Magn Field(T)"=0.0}, {"temperature"=14.473, "lorentzian"={"Amplitude"=0.0, "omega(0)"=0.0, "Gamma"=0.0, "phase"=0.0, "Q"=0.0, "Norm  Ampl"=0.0, "z (inf)"=0.0+0.0i, "4corners"={"z (-pi/2)"=0.0+0.0i, "z(inf)"=0.0+0.0i, "z (pi/2)"=0.0+0.0i, "z center"=0.0+0.0i, "z(0)"=0.0+0.0i, "radius"=0.0}}, "timestamp(min)"=2256.9666666686535, "timestamp"=timestamp(3493863239 s since 1904-01-01), "Magn Field(T)"=0.0}, {"temperature"=14.478, "lorentzian"={"Amplitude"=0.0, "omega(0)"=0.0, "Gamma"=0.0, "phase"=0.0, "Q"=0.0, "Norm  Ampl"=0.0, "z (inf)"=0.0+0.0i, "4corners"={"z (-pi/2)"=0.0+0.0i, "z(inf)"=0.0+0.0i, "z (pi/2)"=0.0+0.0i, "z center"=0.0+0.0i, "z(0)"=0.0+0.0i, "radius"=0.0}}, "timestamp(min)"=2258.3000000044703, "timestamp"=timestamp(3493863319 s since 1904-01-01), "Magn Field(T)"=0.0}, {"temperature"=14.475, "lorentzian"={"Amplitude"=0.0, "omega(0)"=0.0, "Gamma"=0.0, "phase"=0.0, "Q"=0.0, "Norm  Ampl"=0.0, "z (inf)"=0.0+0.0i, "4corners"={"z (-pi/2)"=0.0+0.0i, "z(inf)"=0.0+0.0i, "z (pi/2)"=0.0+0.0i, "z center"=0.0+0.0i, "z(0)"=0.0+0.0i, "radius"=0.0}}, "timestamp(min)"=2259.6166666671634, "timestamp"=timestamp(3493863398 s since 1904-01-01), "Magn Field(T)"=0.0}, {"temperature"=14.47, "lorentzian"={"Amplitude"=0.0, "omega(0)"=0.0, "Gamma"=0.0, "phase"=0.0, "Q"=0.0, "Norm  Ampl"=0.0, "z (inf)"=0.0+0.0i, "4corners"={"z (-pi/2)"=0.0+0.0i, "z(inf)"=0.0+0.0i, "z (pi/2)"=0.0+0.0i, "z center"=0.0+0.0i, "z(0)"=0.0+0.0i, "radius"=0.0}}, "timestamp(min)"=2260.9500000029802, "timestamp"=timestamp(3493863478 s since 1904-01-01), "Magn Field(T)"=0.0}, {"temperature"=14.472, "lorentzian"={"Amplitude"=0.0, "omega(0)"=0.0, "Gamma"=0.0, "phase"=0.0, "Q"=0.0, "Norm  Ampl"=0.0, "z (inf)"=0.0+0.0i, "4corners"={"z (-pi/2)"=0.0+0.0i, "z(inf)"=0.0+0.0i, "z (pi/2)"=0.0+0.0i, "z center"=0.0+0.0i, "z(0)"=0.0+0.0i, "radius"=0.0}}, "timestamp(min)"=2262.2666666656733, "timestamp"=timestamp(3493863557 s since 1904-01-01), "Magn Field(T)"=0.0}, {"temperature"=14.471, "lorentzian"={"Amplitude"=0.0, "omega(0)"=0.0, "Gamma"=0.0, "phase"=0.0, "Q"=0.0, "Norm  Ampl"=0.0, "z (inf)"=0.0+0.0i, "4corners"={"z (-pi/2)"=0.0+0.0i, "z(inf)"=0.0+0.0i, "z (pi/2)"=0.0+0.0i, "z center"=0.0+0.0i, "z(0)"=0.0+0.0i, "radius"=0.0}}, "timestamp(min)"=2263.583333335817, "timestamp"=timestamp(3493863636 s since 1904-01-01), "Magn Field(T)"=0.0}, {"temperature"=14.469, "lorentzian"={"Amplitude"=0.0, "omega(0)"=0.0, "Gamma"=0.0, "phase"=0.0, "Q"=0.0, "Norm  Ampl"=0.0, "z (inf)"=0.0+0.0i, "4corners"={"z (-pi/2)"=0.0+0.0i, "z(inf)"=0.0+0.0i, "z (pi/2)"=0.0+0.0i, "z center"=0.0+0.0i, "z(0)"=0.0+0.0i, "radius"=0.0}}, "timestamp(min)"=2264.916666664183, "timestamp"=timestamp(3493863716 s since 1904-01-01), "Magn Field(T)"=0.0}, {"temperature"=14.466, "lorentzian"={"Amplitude"=0.0, "omega(0)"=0.0, "Gamma"=0.0, "phase"=0.0, "Q"=0.0, "Norm  Ampl"=0.0, "z (inf)"=0.0+0.0i, "4corners"={"z (-pi/2)"=0.0+0.0i, "z(inf)"=0.0+0.0i, "z (pi/2)"=0.0+0.0i, "z center"=0.0+0.0i, "z(0)"=0.0+0.0i, "radius"=0.0}}, "timestamp(min)"=2266.2333333343267, "timestamp"=timestamp(3493863795 s since 1904-01-01), "Magn Field(T)"=0.0}, {"temperature"=14.467, "lorentzian"={"Amplitude"=0.0, "omega(0)"=0.0, "Gamma"=0.0, "phase"=0.0, "Q"=0.0, "Norm  Ampl"=0.0, "z (inf)"=0.0+0.0i, "4corners"={"z (-pi/2)"=0.0+0.0i, "z(inf)"=0.0+0.0i, "z (pi/2)"=0.0+0.0i, "z center"=0.0+0.0i, "z(0)"=0.0+0.0i, "radius"=0.0}}, "timestamp(min)"=2267.5500000044703, "timestamp"=timestamp(3493863874 s since 1904-01-01), "Magn Field(T)"=0.0}, {"temperature"=14.468, "lorentzian"={"Amplitude"=0.0, "omega(0)"=0.0, "Gamma"=0.0, "phase"=0.0, "Q"=0.0, "Norm  Ampl"=0.0, "z (inf)"=0.0+0.0i, "4corners"={"z (-pi/2)"=0.0+0.0i, "z(inf)"=0.0+0.0i, "z (pi/2)"=0.0+0.0i, "z center"=0.0+0.0i, "z(0)"=0.0+0.0i, "radius"=0.0}}, "timestamp(min)"=2268.8833333328366, "timestamp"=timestamp(3493863954 s since 1904-01-01), "Magn Field(T)"=0.0}, {"temperature"=14.463, "lorentzian"={"Amplitude"=0.0, "omega(0)"=0.0, "Gamma"=0.0, "phase"=0.0, "Q"=0.0, "Norm  Ampl"=0.0, "z (inf)"=0.0+0.0i, "4corners"={"z (-pi/2)"=0.0+0.0i, "z(inf)"=0.0+0.0i, "z (pi/2)"=0.0+0.0i, "z center"=0.0+0.0i, "z(0)"=0.0+0.0i, "radius"=0.0}}, "timestamp(min)"=2270.2000000029802, "timestamp"=timestamp(3493864033 s since 1904-01-01), "Magn Field(T)"=0.0}, {"temperature"=14.464, "lorentzian"={"Amplitude"=0.0, "omega(0)"=0.0, "Gamma"=0.0, "phase"=0.0, "Q"=0.0, "Norm  Ampl"=0.0, "z (inf)"=0.0+0.0i, "4corners"={"z (-pi/2)"=0.0+0.0i, "z(inf)"=0.0+0.0i, "z (pi/2)"=0.0+0.0i, "z center"=0.0+0.0i, "z(0)"=0.0+0.0i, "radius"=0.0}}, "timestamp(min)"=2271.5333333313465, "timestamp"=timestamp(3493864113 s since 1904-01-01), "Magn Field(T)"=0.0}, {"temperature"=14.462, "lorentzian"={"Amplitude"=0.0, "omega(0)"=0.0, "Gamma"=0.0, "phase"=0.0, "Q"=0.0, "Norm  Ampl"=0.0, "z (inf)"=0.0+0.0i, "4corners"={"z (-pi/2)"=0.0+0.0i, "z(inf)"=0.0+0.0i, "z (pi/2)"=0.0+0.0i, "z center"=0.0+0.0i, "z(0)"=0.0+0.0i, "radius"=0.0}}, "timestamp(min)"=2272.85000000149, "timestamp"=timestamp(3493864192 s since 1904-01-01), "Magn Field(T)"=0.0}, {"temperature"=14.457, "lorentzian"={"Amplitude"=0.0, "omega(0)"=0.0, "Gamma"=0.0, "phase"=0.0, "Q"=0.0, "Norm  Ampl"=0.0, "z (inf)"=0.0+0.0i, "4corners"={"z (-pi/2)"=0.0+0.0i, "z(inf)"=0.0+0.0i, "z (pi/2)"=0.0+0.0i, "z center"=0.0+0.0i, "z(0)"=0.0+0.0i, "radius"=0.0}}, "timestamp(min)"=2274.166666664183, "timestamp"=timestamp(3493864271 s since 1904-01-01), "Magn Field(T)"=0.0}, {"temperature"=14.457, "lorentzian"={"Amplitude"=0.0, "omega(0)"=0.0, "Gamma"=0.0, "phase"=0.0, "Q"=0.0, "Norm  Ampl"=0.0, "z (inf)"=0.0+0.0i, "4corners"={"z (-pi/2)"=0.0+0.0i, "z(inf)"=0.0+0.0i, "z (pi/2)"=0.0+0.0i, "z center"=0.0+0.0i, "z(0)"=0.0+0.0i, "radius"=0.0}}, "timestamp(min)"=2275.5, "timestamp"=timestamp(3493864351 s since 1904-01-01), "Magn Field(T)"=0.0}, {"temperature"=14.456, "lorentzian"={"Amplitude"=0.0, "omega(0)"=0.0, "Gamma"=0.0, "phase"=0.0, "Q"=0.0, "Norm  Ampl"=0.0, "z (inf)"=0.0+0.0i, "4corners"={"z (-pi/2)"=0.0+0.0i, "z(inf)"=0.0+0.0i, "z (pi/2)"=0.0+0.0i, "z center"=0.0+0.0i, "z(0)"=0.0+0.0i, "radius"=0.0}}, "timestamp(min)"=2276.8166666701436, "timestamp"=timestamp(3493864430 s since 1904-01-01), "Magn Field(T)"=0.0}, {"temperature"=14.45, "lorentzian"={"Amplitude"=0.0, "omega(0)"=0.0, "Gamma"=0.0, "phase"=0.0, "Q"=0.0, "Norm  Ampl"=0.0, "z (inf)"=0.0+0.0i, "4corners"={"z (-pi/2)"=0.0+0.0i, "z(inf)"=0.0+0.0i, "z (pi/2)"=0.0+0.0i, "z center"=0.0+0.0i, "z(0)"=0.0+0.0i, "radius"=0.0}}, "timestamp(min)"=2278.14999999851, "timestamp"=timestamp(3493864510 s since 1904-01-01), "Magn Field(T)"=0.0}, {"temperature"=14.449, "lorentzian"={"Amplitude"=0.0, 
